vi "JSONRPC-GetAsArray.vi"(10 "index":i32, 11 "params":string[](array[string])) -> (3 "output":string[](array[string]))   [LabVIEW 2014]
panel:
  # "GetAsArray"
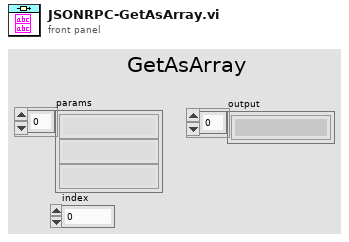
[diagram p1: front panel]
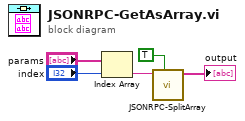
[diagram p0: block diagram]
diagram:
  n1 = Index Array(array="params", index="index") -> (element=w3:string)
  n2 = call "JSONRPC-SplitArray.vi"("unquote strings (false)"=TRUE ("unquote strings (true)"), "input string"=w3) -> ("array"=→"output":string[])  [unwired: 9 in]
